vi "Handle Error.vi"(8 "error in (no error)":errorcluster, 11 "UI ActorTop in":refnum<class "UI_Tree.lvclass">) -> (0 "error out":errorcluster, 2 "stop actor?":bool=TRUE, 3 "UI ActorTop out":refnum<class "UI_Tree.lvclass">)   [LabVIEW 2021, in "UI_Tree.lvlib" / "UI_Tree.lvclass"]
doc: "(<B>Filename</B>: Actor Framework.lvlib:Actor.lvclass:Handle Error.vi)\n\nDefines how the actor handles an error that occurred while processing a message. By default, this method does nothing except stop the actor."
uses:
  UI_Tree.lvclass
  <userlib>/John_Lib/AbstractActorTemplate/AbstractActorTemplate/UIActorTop.lvclass
  UI_Tree.lvclass/UI_Tree.ctl
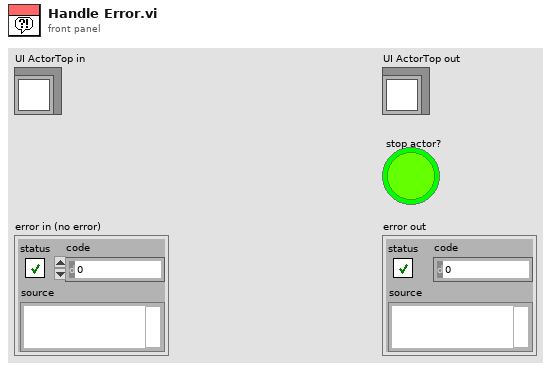
[diagram p1: front panel]
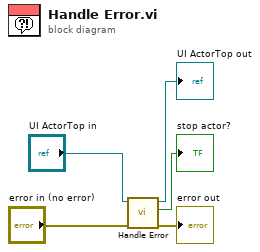
[diagram p0: block diagram]
diagram:
  n1 = call-parent "Handle Error.vi"("error in (no error)"="error in (no error)", "UI ActorTop in"="UI ActorTop in") -> ("error out"=→"error out":errorcluster, "stop actor?"=→"stop actor?":bool, "UI ActorTop out"=→"UI ActorTop out":refnum<class "UI_Tree.lvclass">)  [unwired: 7 in]
